vi "Configure Environment.vi"(8 "error in (no error)":errorcluster, 11 "Test Framework in":refnum<class "Test Framework.lvclass">) -> (0 "error out":errorcluster, 3 "Test Framework out":refnum<class "Test Framework.lvclass">)   [LabVIEW 2020, in "Test Framework.lvclass"]
doc: "Configures the temperature and voltage for the tests"
uses:
  Test Framework.lvclass
  Controls/Temperature and voltage modes.ctl
  Controls/Temperature and voltage array.ctl
  Controls/PSU setting UI.ctl
  Test Framework.lvclass/Test Framework.ctl
  Instruments/Power Supply/Power Supply.lvclass
  C:/Sandbox/RF Bench/Source Code/WiSpry Test Framework/Instruments/Instrument.lvclass
  Instruments/Power Supply/Controls/Source mode.ctl
  Instruments/Instrument.lvclass/Instrument.ctl
  Instruments/Power Supply/Power Supply.lvclass/Power Supply.ctl
  Instruments/Instrument.lvclass
panel:
  in  "Cancel Button":bool
  out "Temperature (C)":dbl(slide) scale=0.0..100.0
  in  "Voltage label":string="Voltage (V)      Voltage sweep (V)        Current limit (A)"
  in  "Current label":string="Current (A)     Current sweep (A)        Voltage limit (V)"
  in  "Available PSU's":T1[](array[typedef])=[{"Enabled"=FALSE, "Source"=enum."Voltage", "Drive (V/A)"=0.0, "Sweep (V/A)"="3.3", "Limit (A/V)"=0.1, "PSU Alias"="PSU2", "PSU info"={"ID"="Agilent Technologies, E3647A", "Address"="GPIB0::5::INSTR", "Channel"=1}}]
  in  "Soak time (min)":dbl
  in  "Temperature (C)":string="25"
  in  "Done Button":bool
  in  "Temperature control array":T2
  in  "Control mode":T3
  # "e.g. \"25,85,-40\""
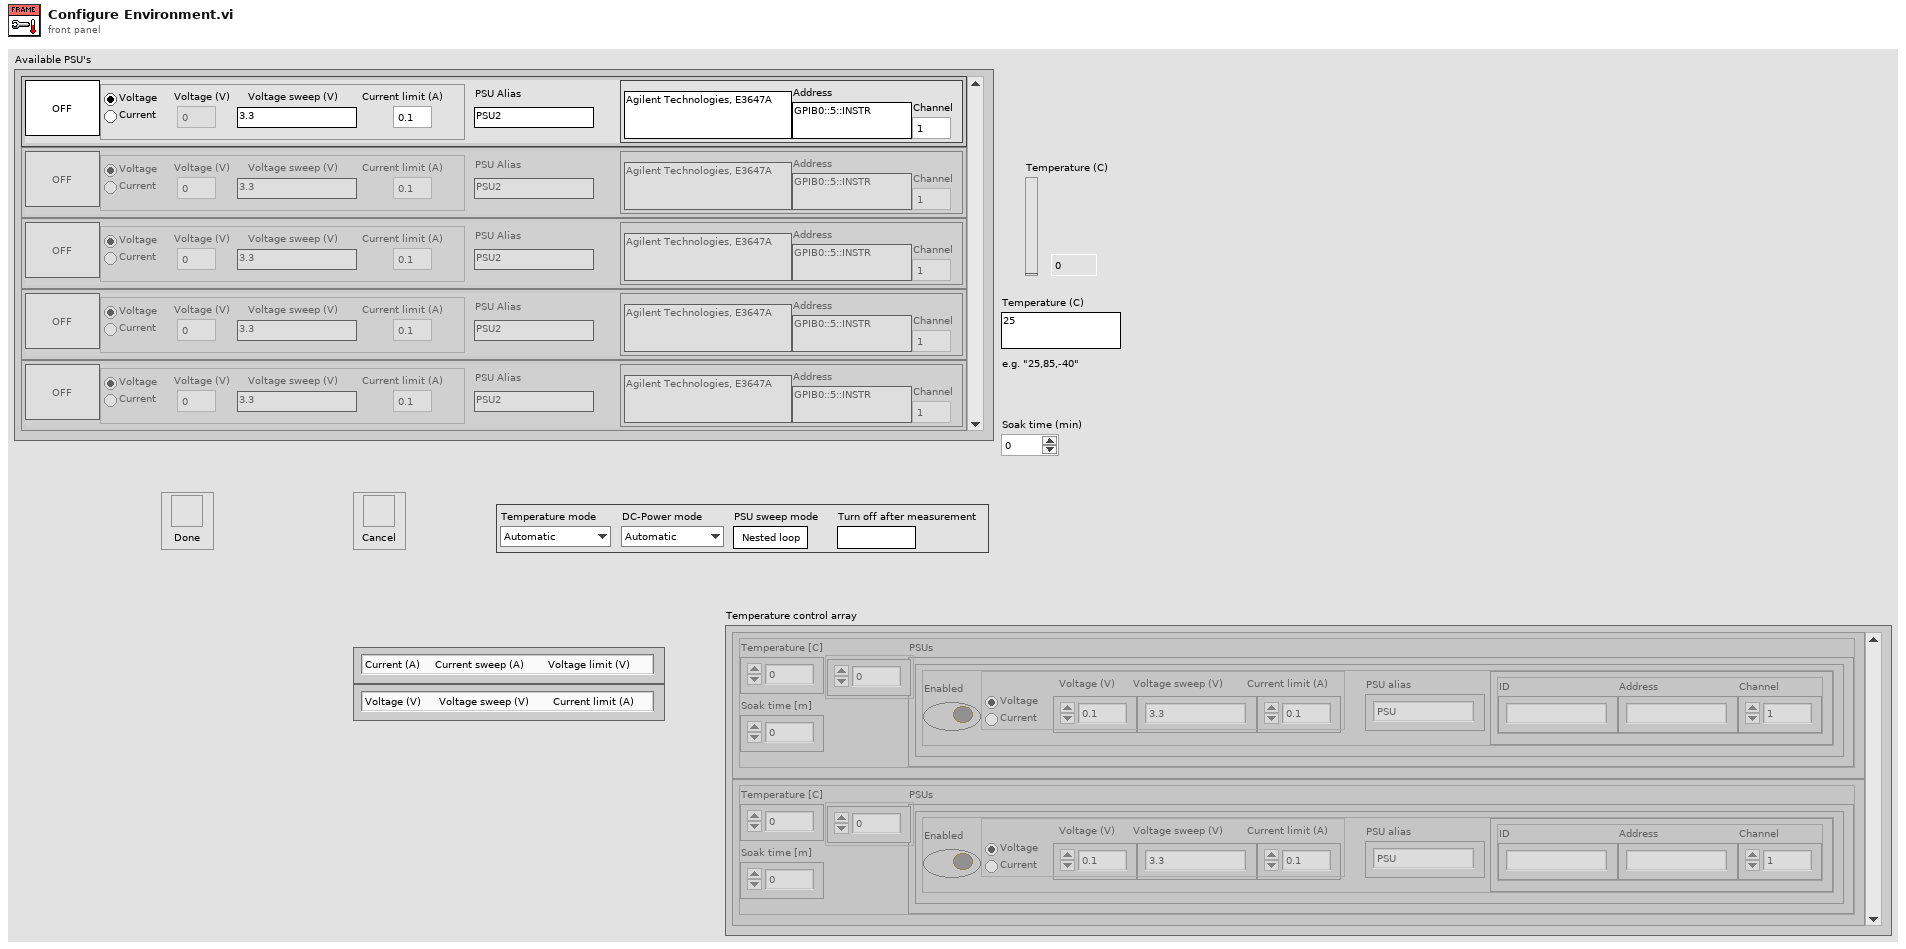
[diagram p1: front panel]
types:
  T1 = typedef "Test Framework.lvclass/PSU setting UI.ctl" = cluster{"Enabled":bool, "Source":enum32{"Voltage", "Current"}, "Drive (V/A)":dbl, "Sweep (V/A)":string, "Limit (A/V)":dbl, "PSU Alias":string, "PSU info":cluster{"ID":string, "Address":string, "Channel":u8}}
  T2 = typedef "Test Framework.lvclass/Temperature and voltage array.ctl" = cluster{"Temperature [C]":dbl, "Soak time [m]":dbl, "PSUs":cluster{"Enabled":bool, "Source":enum32{"Voltage", "Current"}, "Drive (V/A)":dbl, "Sweep (V/A)":string, "Limit (A/V)":dbl, "PSU alias":string, "PSU info":cluster{"ID":string, "Address":string, "Channel":u8}}[]}[]
  T3 = typedef "Test Framework.lvclass/Temperature and voltage modes.ctl" = cluster{"Temperature mode":enum16{"Automatic", "Manual", "Off"}, "DC-Power mode":enum16{"Automatic", "Manual", "Off"}, "PSU sweep mode":bool, "Turn off after measurement":bool}
  T4 = typedef "Power Supply.lvclass/Source mode.ctl" = enum32{"Voltage", "Current"}
  T5 = cluster{"Temperature control array":T2, "Temperature mode":T3}
  T6 = cluster{"Instrument Name":string, "Instrument.lvclass":refnum<class "Instrument.lvclass">, "Reference":bool}[]
  T7 = typedef "Instrument.lvclass/Interface String Cluster.ctl" = cluster{"Interface":string, "IDN string":string, "Instance":i32}
  T8 = cluster{"Temperature [C]":dbl, "Soak time [m]":dbl, "PSUs":cluster{"Enabled":bool, "Source":enum32{"Voltage", "Current"}, "Drive (V/A)":dbl, "Sweep (V/A)":string, "Limit (A/V)":dbl, "PSU alias":string, "PSU info":cluster{"ID":string, "Address":string, "Channel":u8}}[]}
  T9 = cluster{"Instrument Name":string, "Instrument.lvclass":refnum<class "Instrument.lvclass">, "Reference":bool}
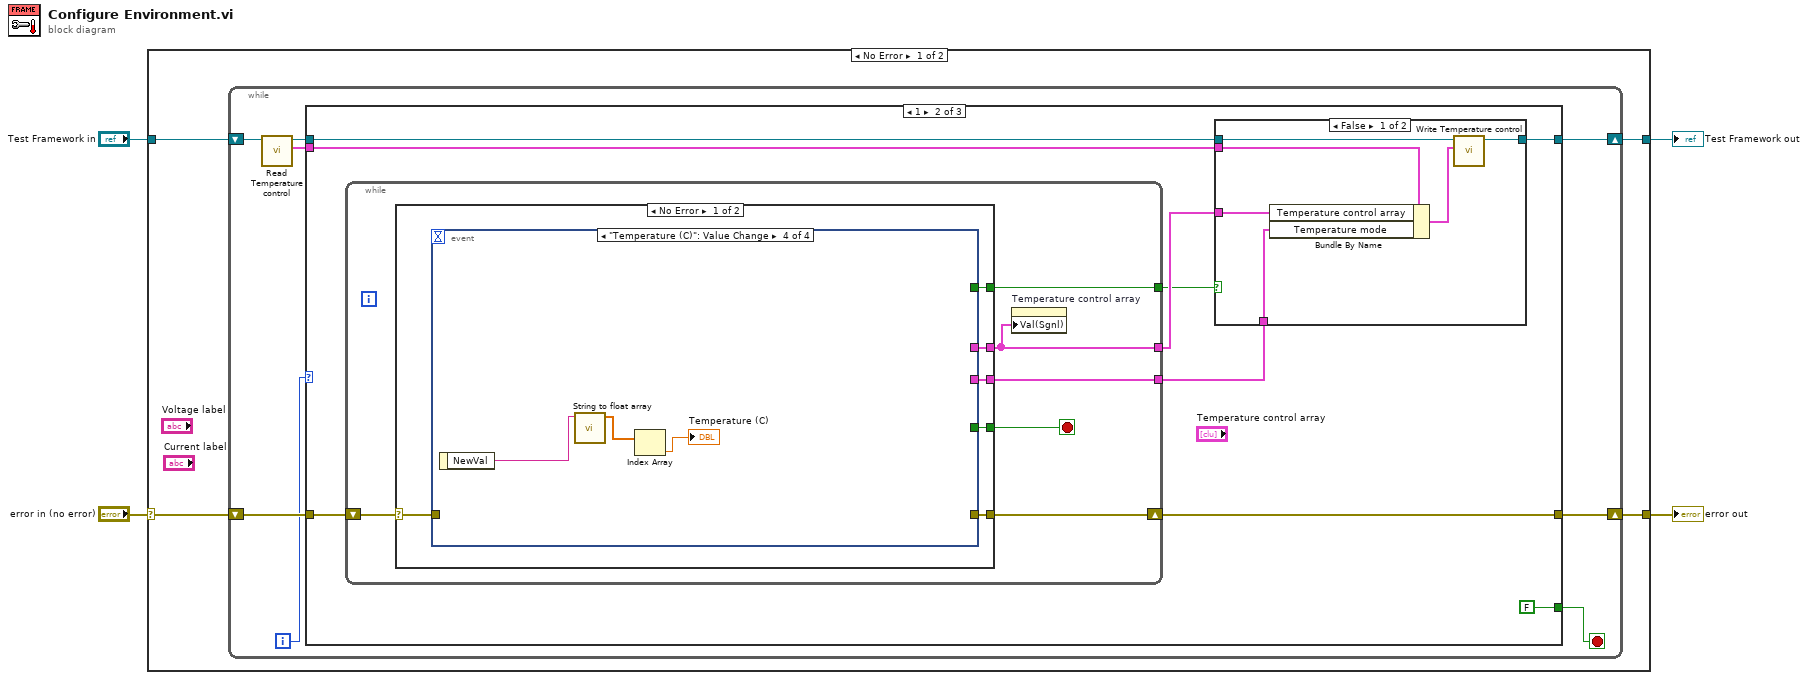
[diagram p0: block diagram]
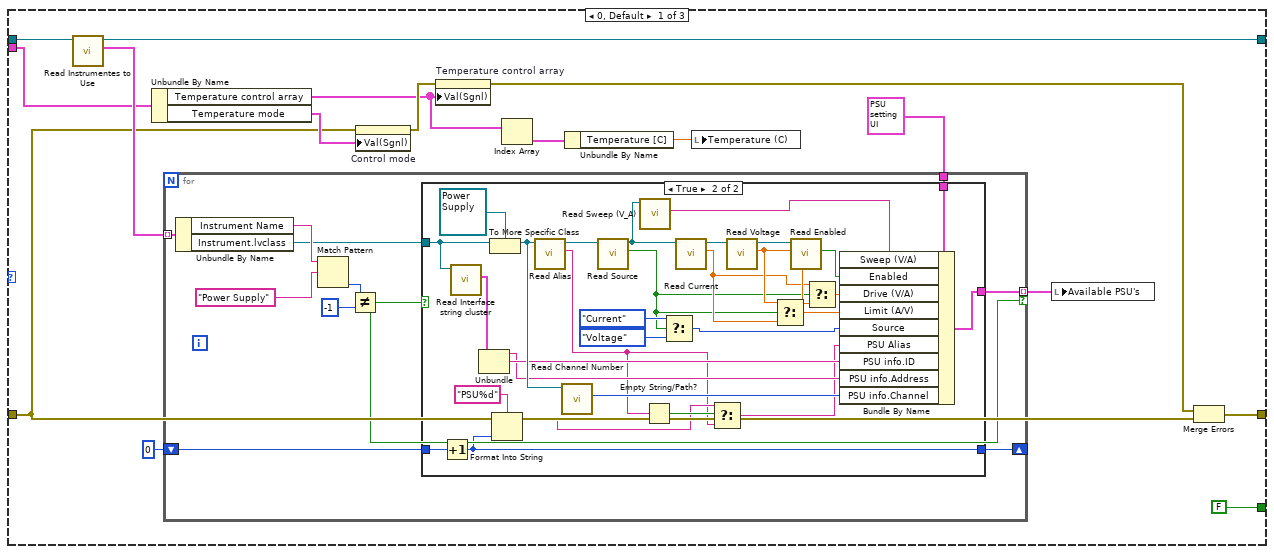
[diagram p2: hidden frame]
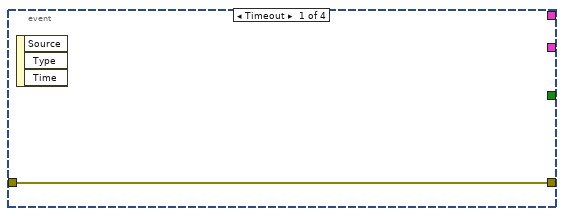
[diagram p5: hidden frame]
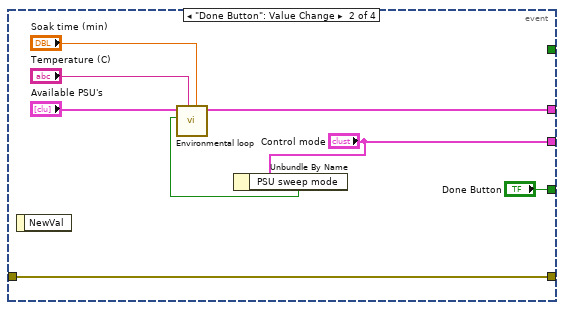
[diagram p6: hidden frame]
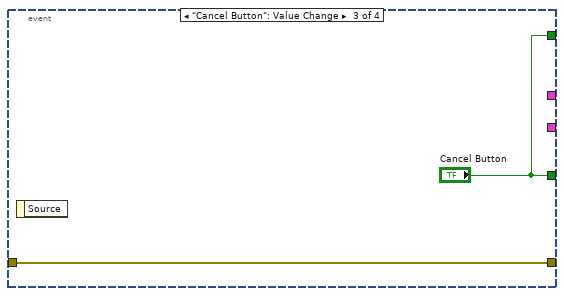
[diagram p7: hidden frame]
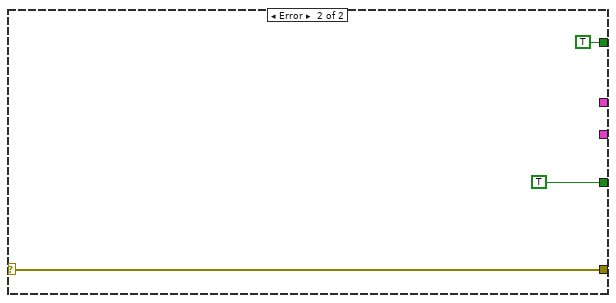
[diagram p8: hidden frame]
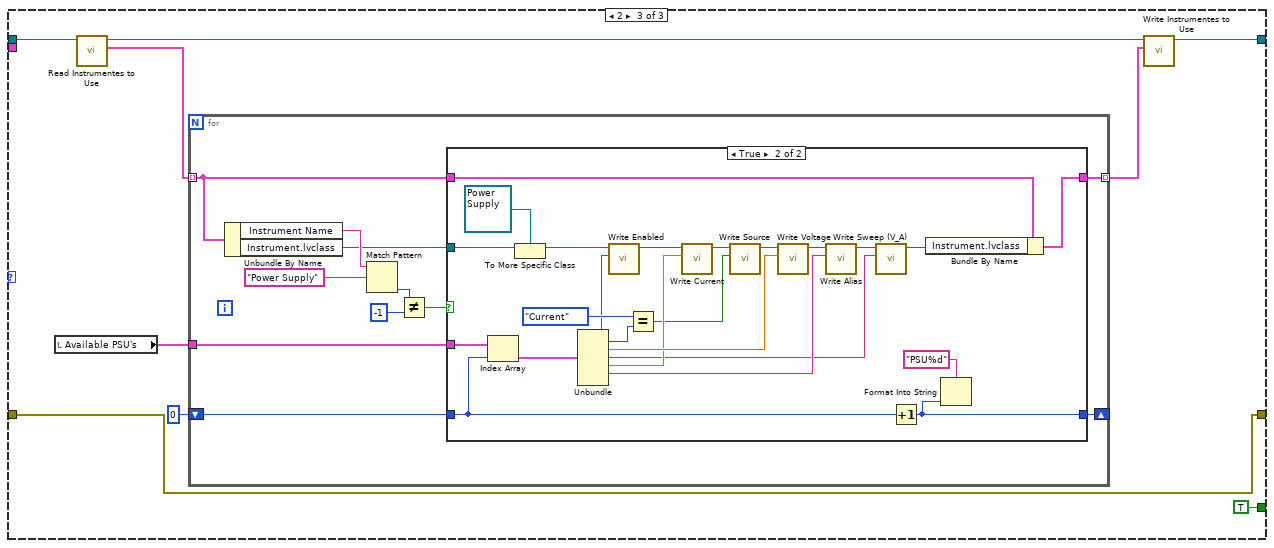
[diagram p9: hidden frame]
diagram:
  n1 = case shown="No Error" "error in (no error)" {
    selector: "error in (no error)" -> [w6 w168]
    tunnel: [w8 w168] -> w3
    tunnel: [w7 w167] -> w2
    tunnel: "Test Framework in" -> [w5 w167]
    frame No Error {
      n2 = while {
        shift-right: [w15] -> w8
        shift-left: w6 -> [w16]
        shift-right: [w10] -> w7
        shift-left: w5 -> [w14]
        i -> [w13]
        stop <- w9 stop-if-true
        n3 = call-dynamic "Read Temperature control.vi"("Test Framework in"=w14) -> ("Temperature control"=w12:T5, "Test Framework out"=w11:refnum<class "Test Framework.lvclass">)  [unwired: 9 in]
        n4 = case shown="1" w13 {
          tunnel: w16 -> [w29 w84 w122]
          tunnel: [w27 w83 w122] -> w15
          tunnel: w11 -> [w26 w82 w127]
          tunnel: [w24 w79 w129] -> w10
          tunnel: w12 -> [w25 w78 _]
          tunnel: [FALSE FALSE TRUE] -> w9
          frame 0, Default {
            n5 = call "Read Instrumentes to Use.vi"("Test Framework in"=w26) -> ("Instrumentes to Use"=w32:T6, "Test Framework out"=w24:refnum<class "Test Framework.lvclass">)  [unwired: 9 in]
            n6 = Unbundle By Name(w25) -> ("Temperature control array"=w19:T2, "Temperature mode"=w31:T3)
            n7 = for {
              tunnel: w32 -> [w43] mode=indexing
              tunnel: T1 {"Enabled"=FALSE, "Source"=enum."Voltage", "Drive (V/A)"=3.3, "Sweep (V/A)"="3.3", "Limit (A/V)"=0.1, "PSU Alias"="Vdd", "PSU info"={"ID"="", "Address"="", "Channel"=0}} ("PSU") -> [w38]
              tunnel: [w36] -> w22 mode=indexing if=w35
              shift-right: [w33] -> _
              shift-left: 0 -> [w34]
              n8 = Unbundle By Name(w43) -> ("Instrument Name"=w42:string, "Instrument.lvclass"=w37:refnum<class "Instrument.lvclass">)
              n9 = Match Pattern(string=w42, regular expression="Power Supply" ("Instrument Name")) -> (offset past match=w40:i32)  [unwired: 1 in, 3 out]
              n10 = Not Equal?(x=w40, y=-1) -> (x != y?=w35:bool)
              n11 = case shown="True" w35 {
                tunnel: w38 -> [w45 w75]
                tunnel: w37 -> [_ w64]
                tunnel: [w45 w65] -> w36
                tunnel: w34 -> [w44 w58]
                tunnel: [w44 w57] -> w33
                frame False {
                }
                frame True {
                  n12 = Increment(x=w58) -> (x+1=w57:i32)
                  n13 = call "Read Interface string cluster.vi"("Instrument in"=w64) -> ("Interface sting cluster"=w62:T7)  [unwired: 9 in, 1 out]
                  n14 = Unbundle(w62) -> ("Interface"=w60:string, "IDN string"=w61:string)  [unwired: 1 out]
                  n15 = To More Specific Class(target class=refnum<class "Power Supply.lvclass"> refnum ("Power Supply out"), reference=w64) -> (specific class reference=w63:refnum<class "Power Supply.lvclass">)  [unwired: 1 in, 1 out]
                  n16 = Format Into String(format string="PSU%d", w57) -> (resulting string=w54:string)  [unwired: 2 in, 1 out]
                  n17 = call-dynamic "Read Alias.vi"("Power Supply in"=w63) -> ("Alias"=w53:string, "Power Supply out"=w73:refnum<class "Power Supply.lvclass">)  [unwired: 9 in]
                  n18 = call "Read Channel Number.vi"("Power Supply in"=w63) -> ("Channel Number"=w59:u8)  [unwired: 9 in, 1 out]
                  n19 = call-dynamic "Read Source.vi"("Power Supply in"=w73) -> ("Source"=w66:bool, "Power Supply out"=w47:refnum<class "Power Supply.lvclass">)  [unwired: 9 in]
                  n20 = call-dynamic "Read Sweep (V_A).vi"("Power Supply in"=w47) -> ("Sweep (V/A)"=w48:string)  [unwired: 9 in, 1 out]
                  n21 = Empty String/Path?(string/path=w53) -> (empty?=w55:bool)
                  n22 = Select(t=Source_mode."Current" ("Source"), s=w66, f=Source_mode."Voltage" ("Source")) -> (s? t:f=w46:T4)
                  n23 = call "Read Current.vi"("Power Supply in"=w47) -> ("Current"=w67:dbl, "Power Supply out"=w72:refnum<class "Power Supply.lvclass">)  [unwired: 9 in]
                  n24 = Select(t=w54, s=w55, f=w53) -> (s? t:f=w52:string)
                  n25 = call "Read Voltage.vi"("Power Supply in"=w72) -> ("Voltage"=w68:dbl, "Power Supply out"=w50:refnum<class "Power Supply.lvclass">)  [unwired: 9 in]
                  n26 = Select(t=w68, s=w66, f=w67) -> (s? t:f=w69:dbl)
                  n27 = call-dynamic "Read Enabled.vi"("Power Supply in"=w50) -> ("Enabled"=w49:bool)  [unwired: 9 in, 1 out]
                  n28 = Select(t=w67, s=w66, f=w68) -> (s? t:f=w70:dbl)
                  n29 = Bundle By Name(cluster=w75, "Sweep (V/A)"=w48, "Enabled"=w49, "Drive (V/A)"=w70, "Limit (A/V)"=w69, "Source"=w46, "PSU Alias"=w52, "PSU info.ID"=w61, "PSU info.Address"=w60, "PSU info.Channel"=w59) -> (w65:T1)
                }
              }
            }
            n30 = property on="Control mode" class="Clust"(error in=w29, "Val(Sgnl)"=w31) -> (error out=w28:errorcluster)  [unwired: 1 in, 1 out]
            n31 = property on="Temperature control array" class="Arr (strict)"(error in=w28, "Val(Sgnl)"=w19) -> (error out=w30:errorcluster)  [unwired: 1 in, 1 out]
            n32 = Index Array(array=w19) -> (element=w18:T8)  [unwired: 1 in]
            n33 = Unbundle By Name(w18) -> ("Temperature [C]"=w17:dbl)
            n34 = local write "Temperature (C)"(w17) -> ()
            n35 = local write "Available PSU's"(w22) -> ()
            n36 = Merge Errors(w30, w29) -> (w27:errorcluster)
          }
          frame 1 {
            n37 = while {
              shift-right: [w95] -> w83
              shift-left: w84 -> [w96]
              tunnel: [w94] -> w80
              tunnel: [w93] -> w81
              tunnel: [w92] -> w76
              stop <- w97 stop-if-true
              n38 = case shown="No Error" w96 {
                selector: w96 -> [w101 w119]
                tunnel: [w103 TRUE ("Done Button")] -> w97
                tunnel: [w102 w119] -> w95
                tunnel: [w99 _] -> w93
                tunnel: [w100 _] -> w94
                tunnel: [w98 TRUE ("Cancel Button")] -> w92
                frame No Error {
                  n39 = event shown="[3] \"Temperature (C)\": Value Change" {
                    selector: _ -> [_ _ _ _]
                    dyn-events: _ -> [_ _ _ _]
                    timeout: _ -> [_ _ _ _]
                    tunnel: [_ "Done Button" "Cancel Button" _] -> w103
                    tunnel: [w104 w111 w114 _] -> w102
                    tunnel: w101 -> [w104 w111 w114 _]
                    tunnel: [_ "Control mode" _ _] -> w100
                    tunnel: [_ w107 _ _] -> w99
                    tunnel: [_ _ "Cancel Button" _] -> w98
                    event Timeout {
                      n40 = event-data() -> ()  [unwired: 1 in, 3 out]
                    }
                    event "Done Button": Value Change {
                      n41 = event-data() -> ()  [unwired: 1 in, 1 out]
                      n42 = Unbundle By Name("Control mode") -> ("PSU sweep mode"=w105:bool)
                      n43 = call "Environmental loop.vi"("Soak time (min)"="Soak time (min)", "Temperature (C)"="Temperature (C)", "Synchronized step"=w105, "Available PSU's"="Available PSU's") -> ("Temperature control array"=w107:T2)  [unwired: 7 in]
                    }
                    event "Cancel Button": Value Change {
                      n44 = event-data() -> ()  [unwired: 1 in, 1 out]
                    }
                    event "Temperature (C)": Value Change {
                      n45 = event-data() -> ("NewVal"=w117:string)  [unwired: 1 in]
                      n46 = call "String to float array.vi"("String"=w117) -> ("Array - Numeric"=w116:dbl[])  [unwired: 9 in, 1 out]
                      n47 = Index Array(array=w116) -> (element=→"Temperature (C)":dbl)  [unwired: 1 in]
                    }
                  }
                }
                frame Error {
                }
              }
              n48 = property on="Temperature control array" class="Arr (strict)"("Val(Sgnl)"=w93) -> ()  [unwired: 2 in, 2 out]
            }
            n49 = case shown="False" w76 {
              tunnel: w82 -> [w90 w91]
              tunnel: w81 -> [w89 _]
              tunnel: w80 -> [w88 _]
              tunnel: [w86 w91] -> w79
              tunnel: w78 -> [w85 _]
              frame False {
                n50 = Bundle By Name(cluster=w85, "Temperature control array"=w89, "Temperature mode"=w88) -> (w87:T5)
                n51 = call-dynamic "Write Temperature control.vi"("Temperature control"=w87, "Test Framework in"=w90) -> ("Test Framework out"=w86:refnum<class "Test Framework.lvclass">)  [unwired: 9 in]
              }
              frame True {
                # "Canceled"
              }
            }
          }
          frame 2 {
            n52 = local read "Available PSU's"() -> (w124:T1[])
            n53 = call "Read Instrumentes to Use.vi"("Test Framework in"=w127) -> ("Instrumentes to Use"=w125:T6, "Test Framework out"=w128:refnum<class "Test Framework.lvclass">)  [unwired: 9 in]
            n54 = for {
              tunnel: w125 -> [w131] mode=indexing
              shift-right: [w133] -> _
              shift-left: 0 -> [w134]
              tunnel: w124 -> [w132]
              tunnel: [w130] -> w123 mode=indexing
              n55 = Unbundle By Name(w131) -> ("Instrument Name"=w140:string, "Instrument.lvclass"=w136:refnum<class "Instrument.lvclass">)
              n56 = Match Pattern(string=w140, regular expression="Power Supply" ("Instrument Name")) -> (offset past match=w138:i32)  [unwired: 1 in, 3 out]
              n57 = Not Equal?(x=w138, y=-1) -> (x != y?=w135:bool)
              n58 = case shown="True" w135 {
                tunnel: w136 -> [_ w165]
                tunnel: w134 -> [w142 w161]
                tunnel: [w142 w164] -> w133
                tunnel: w132 -> [_ w162]
                tunnel: w131 -> [w141 w157]
                tunnel: [w141 w156] -> w130
                frame False {
                }
                frame True {
                  n59 = Index Array(array=w162, index=w161) -> (element=w155:T1)
                  n60 = To More Specific Class(target class=refnum<class "Power Supply.lvclass"> refnum ("Power Supply out"), reference=w165) -> (specific class reference=w147:refnum<class "Power Supply.lvclass">)  [unwired: 1 in, 1 out]
                  n61 = Unbundle(w155) -> ("Enabled"=w148:bool, "Source"=w150:enum32{"Voltage", "Current"}, "Drive (V/A)"=w154:dbl, "Sweep (V/A)"=w143:string, "Limit (A/V)"=w153:dbl, "PSU Alias"=w152:string)  [unwired: 1 out]
                  n62 = call-dynamic "Write Enabled.vi"("Enabled"=w148, "Power Supply in"=w147) -> ("Power Supply out"=w146:refnum<class "Power Supply.lvclass">)  [unwired: 9 in]
                  n63 = Equal?(x=Source_mode."Current" ("Source"), y=w150) -> (x = y?=w149:bool)
                  n64 = call "Write Current.vi"("Current"=w153, "Power Supply in"=w146) -> ("Power Supply out"=w160:refnum<class "Power Supply.lvclass">)  [unwired: 9 in]
                  n65 = call-dynamic "Write Source.vi"("Source"=w149, "Power Supply in"=w160) -> ("Power Supply out"=w159:refnum<class "Power Supply.lvclass">)  [unwired: 9 in]
                  n66 = call "Write Voltage.vi"("Voltage"=w154, "Power Supply in"=w159) -> ("Power Supply out"=w158:refnum<class "Power Supply.lvclass">)  [unwired: 9 in]
                  n67 = call-dynamic "Write Alias.vi"("Alias"=w152, "Power Supply in"=w158) -> ("Power Supply out"=w145:refnum<class "Power Supply.lvclass">)  [unwired: 9 in]
                  n68 = call-dynamic "Write Sweep (V_A).vi"("Sweep (V/A)"=w143, "Power Supply in"=w145) -> ("Power Supply out"=w144:refnum<class "Power Supply.lvclass">)  [unwired: 9 in]
                  n69 = Increment(x=w161) -> (x+1=w164:i32)
                  n70 = Bundle By Name(cluster=w157, "Instrument.lvclass"=w144) -> (w156:T9)
                  n71 = Format Into String(format string="PSU%d", w164) -> ()  [unwired: 2 in, 2 out]
                }
              }
            }
            n72 = call "Write Instrumentes to Use.vi"("Instruments to Use"=w123, "Test Framework in"=w128) -> ("Test Framework out"=w129:refnum<class "Test Framework.lvclass">)  [unwired: 9 in]
          }
        }
      }
    }
    frame Error {
    }
  }
  "error out" <- w3
  "Test Framework out" <- w2
